vi "Test camera live.vi"(8 "Gain":i32 min=100 max=2000 step=1, 9 "Exposure time (ms)":dbl=100.0 min=1.0 max=10000.0 step=1.0) -> (2 "Image out":T1(plugin-control))   [LabVIEW 2017]
uses:
  C:/Program Files/National Instruments/LabVIEW 2017/instr.lib/IDS/ueye.NET/uEyeDotNet.dll
panel:
  in  "Width":i32=2456
  in  "Height":i32=2054
  in  "PosY":i32
  in  "PosX":i32
  out "Actual frame time (ms)":u32
  in  "stop":bool
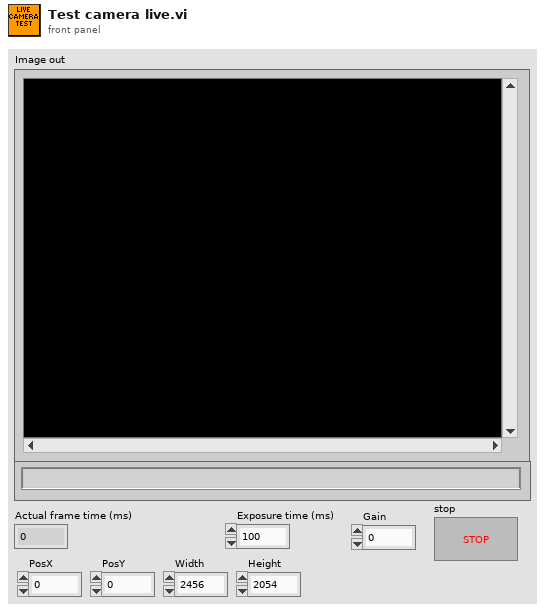
[diagram p1: front panel]
types:
  T1 = typedef "IMAQ Image.ctl" = refnum<image>
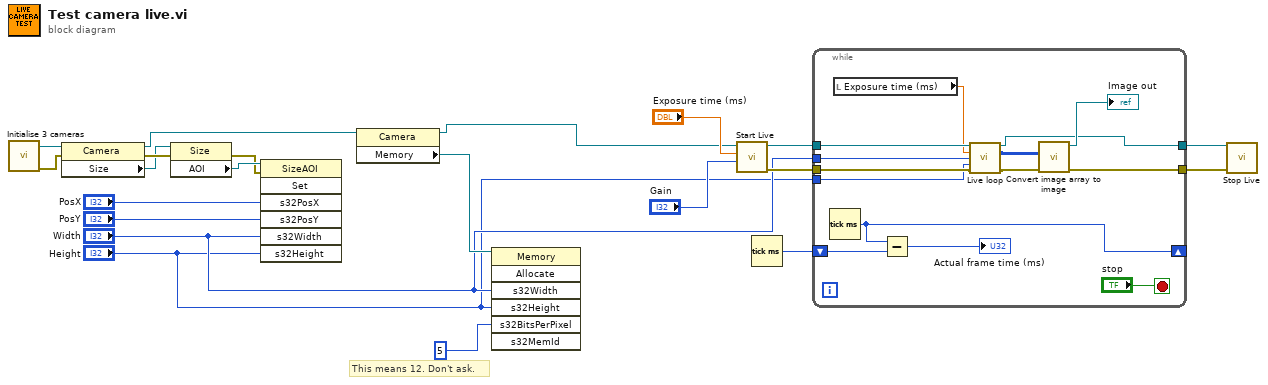
[diagram p0: block diagram]
diagram:
  # "This means 12. Don't ask."
  n1 = call "Initialise 3 cameras.vi"() -> ("Error Out"=w9:errorcluster, "Red camera ref"=w12:refnum<k24>)  [unwired: 8 in, 2 out]
  n2 = property class="Camera"(reference=w12, error in=w9) -> (reference out=w6:refnum<k24>, error out=w14:errorcluster, "Size"=w13:refnum<k24>)
  n3 = property class="Size"(reference=w13, error in=w14) -> (error out=w10:errorcluster, "AOI"=w11:refnum<k24>)  [unwired: 1 out]
  n4 = invoke class="SizeAOI" method="Set"(reference=w11, error in=w10, "s32PosX"="PosX", "s32PosY"="PosY", "s32Width"="Width", "s32Height"="Height") -> ()  [unwired: 1 in, 7 out]
  n5 = property class="Camera"(reference=w6) -> (reference out=w5:refnum<k24>, "Memory"=w4:refnum<k24>)  [unwired: 1 in, 1 out]
  n6 = invoke class="Memory" method="Allocate"(reference=w4, "s32Width"="Width", "s32Height"="Height", "s32BitsPerPixel"=5) -> ()  [unwired: 3 in, 7 out]
  n7 = call "Start Live.vi"("Gain in"="Gain", "Exposure time (ms)"="Exposure time (ms)", "Camera reference in"=w5) -> ("Error Out"=w16:errorcluster, "Camera reference out"=w15:refnum<k24>)  [unwired: 6 in]
  n8 = Tick Count (ms)() -> (millisecond timer value=w17:u32)
  n9 = while {
    tunnel: [w34] -> w19
    tunnel: [w28] -> w18
    tunnel: w15 -> [w25]
    tunnel: w16 -> [w26]
    shift-right: [w31] -> _
    shift-left: w17 -> [w32]
    tunnel: "Width" -> [w23]
    tunnel: "Height" -> [w22]
    stop <- "stop" stop-if-true
    n10 = Tick Count (ms)() -> (millisecond timer value=w31:u32)
    n11 = local read "Exposure time (ms)"() -> (w24:dbl)
    n12 = Subtract(x=w31, y=w32) -> (x-y=→"Actual frame time (ms)":u32)
    n13 = call "Live loop.vi"("Camera reference in"=w25, "Exposure (ms)"=w24, "Width"=w23, "Height"=w22, "Error In"=w26) -> ("Camera reference out"=w28:refnum<k24>, "Image Array"=w29:u16[][], "Error Out"=w27:errorcluster)  [unwired: 8 in]
    n14 = call "Convert image array to image.vi"("Error In"=w27, "Array"=w29) -> ("error out"=w34:errorcluster, "Image Out"=→"Image out":T1)  [unwired: 7 in]
  }
  n15 = call "Stop Live.vi"("Camera reference in"=w18, "Error In"=w19) -> ()  [unwired: 16 in, 2 out]
